vi "SsFileName.vi"(8 "error in (no error)":errorcluster, 10 "Time":string, 11 "Function Params":dbl[][](array[numeric])) -> (0 "error out":errorcluster, 3 "FileName":string)   [LabVIEW 2018, in "AnalysisPlugins.lvlib" / "PmuAnalysis.lvclass"]
uses:
  PmuAnalysis.lvclass
  FGen/MemberClasses/PmuTestFunctions/Typedefs/eParamIdx.ctl
  FGen/MemberClasses/PmuTestFunctions/PmuTestFunctions.lvclass
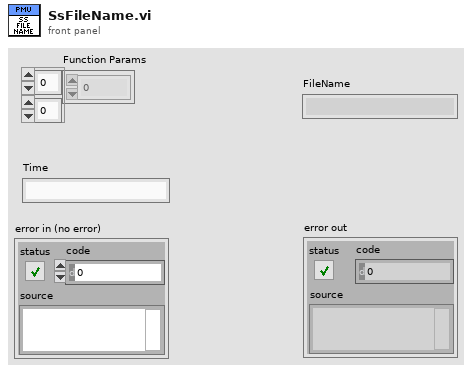
[diagram p1: front panel]
types:
  T1 = typedef "Functions.lvlib/PmuTestFunctions.lvclass/eParamIdx.ctl" = enum16{"Xm", "Fin", "Ps", "Fh", "Ph", "Kh", "Fa", "Ka", "Fx", "Kx", "Rf", "KaS", "KxS", "KfS", "KrS"}
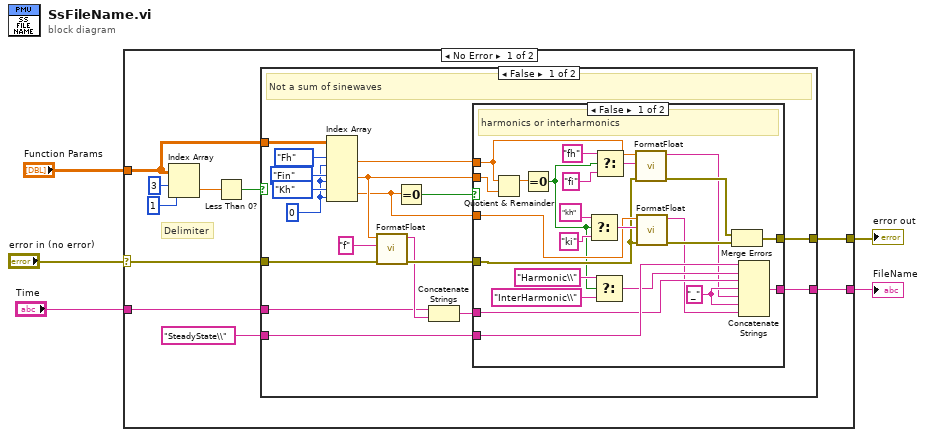
[diagram p0: block diagram]
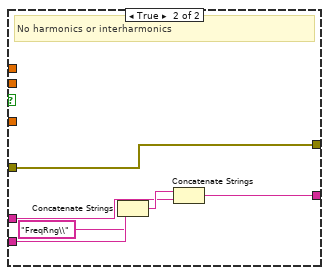
[diagram p2: hidden frame]
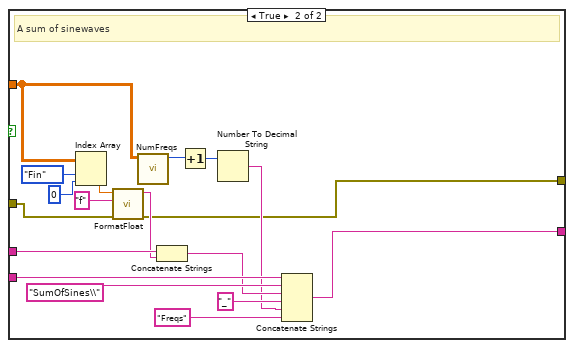
[diagram p3: hidden frame]
diagram:
  n1 = case shown="No Error" "error in (no error)" {
    selector: "error in (no error)" -> [w9 w82]
    tunnel: "Function Params" -> [w10 _]
    tunnel: "Time" -> [w11 _]
    tunnel: [w8 _] -> w2
    tunnel: [w7 w82] -> w1
    frame No Error {
      # "Delimiter"
      n2 = Index Array(array=w10, index (row)=3, index (col)=1 ("disabled index (col)")) -> (element=w13:dbl)
      n3 = Less Than 0?(x=w13) -> (x < 0?=w12:bool)
      n4 = case shown="False" w12 {
        tunnel: w11 -> [w19 w76]
        tunnel: w10 -> [w33 w64]
        tunnel: w9 -> [w27 w77]
        tunnel: [w18 w67] -> w8
        tunnel: [w17 w66] -> w7
        tunnel: "SteadyState\\" -> [w16 w74]
        frame False {
          w29 = 0
          # "Not a sum of sinewaves"
          n5 = Index Array(array=w33, index (row) #1=eParamIdx."Fh" ("eParamIdx"), index (col) #1=w29, index (row) #2=eParamIdx."Fin" ("eParamIdx"), index (col) #2=w29, index (row) #3=eParamIdx."Kh" ("eParamIdx"), index (col) #3=w29) -> (element #1=w24:dbl, element #2=w25:dbl, element #3=w23:dbl)
          n6 = call "FormatFloat.vi"("error in (no error)"=w27, "replace string (\".\")"="f" ("replace string (\".\")"), "float"=w25) -> ("error out"=w22:errorcluster, "string"=w21:string)  [unwired: 7 in]
          n7 = Equal To 0?(x=w23) -> (x = 0?=w26:bool)
          n8 = Concatenate Strings(w19, w21) -> (w20:string)
          n9 = case shown="False" w26 {
            tunnel: w22 -> [w43 w58]
            tunnel: w20 -> [w37 w60]
            tunnel: w16 -> [w42 w63]
            tunnel: [w50 w59] -> w18
            tunnel: [w56 w58] -> w17
            tunnel: w24 -> [w49 _]
            tunnel: w25 -> [w48 _]
            tunnel: w23 -> [w44 _]
            frame False {
              w35 = "_" ("string")
              # "harmonics or interharmonics"
              n10 = Quotient & Remainder(x=w49, y=w48) -> (x-y*floor(x/y)=w47:dbl)  [unwired: 1 out]
              n11 = Equal To 0?(x=w47) -> (x = 0?=w39:bool)
              n12 = Select(t="kh" ("replace string (\".\")"), s=w39, f="ki" ("replace string (\".\")")) -> (s? t:f=w53:string)
              n13 = Select(t="Harmonic\\", s=w39, f="InterHarmonic\\") -> (s? t:f=w38:string)
              n14 = Select(t="fh" ("replace string (\".\")"), s=w39, f="fi" ("replace string (\".\")")) -> (s? t:f=w57:string)
              n15 = call "FormatFloat.vi"("error in (no error)"=w43, "replace string (\".\")"=w57, "float"=w49) -> ("error out"=w55:errorcluster, "string"=w34:string)  [unwired: 7 in]
              n16 = call "FormatFloat.vi"("error in (no error)"=w43, "replace string (\".\")"=w53, "float"=w44) -> ("error out"=w54:errorcluster, "string"=w36:string)  [unwired: 7 in]
              n17 = Merge Errors(w55, w54) -> (w56:errorcluster)
              n18 = Concatenate Strings(w42, w38, w37, w35, w34, w35, w36) -> (w50:string)
            }
            frame True {
              # "No harmonics or interharmonics"
              n19 = Concatenate Strings(w63, "FreqRng\\") -> (w61:string)
              n20 = Concatenate Strings(w61, w60) -> (w59:string)
            }
          }
        }
        frame True {
          # "A sum of sinewaves"
          n21 = Index Array(array=w64, index (row)=eParamIdx."Fin" ("eParamIdx"), index (col)=0 ("disabled index (col)")) -> (element=w79:dbl)
          n22 = call "FormatFloat.vi"("error in (no error)"=w77, "replace string (\".\")"="f" ("replace string (\".\")"), "float"=w79) -> ("error out"=w66:errorcluster, "string"=w75:string)  [unwired: 7 in]
          n23 = call "NumFreqs.vi"("TestParams"=w64) -> ("NumFreqs"=w65:i32)  [unwired: 6 in]
          n24 = Concatenate Strings(w76, w75) -> (w72:string)
          n25 = Increment(x=w65) -> (x+1=w68:i32)
          n26 = Number To Decimal String(number=w68) -> (decimal integer string=w70:string)  [unwired: 1 in]
          n27 = Concatenate Strings(w74, "SumOfSines\\", w72, "_" ("string"), w70, "Freqs" ("string")) -> (w67:string)
        }
      }
    }
    frame Error {
    }
  }
  "error out" <- w1
  "FileName" <- w2
